vi "Exit Initialize (User).vi"(8 "error in":errorcluster, 11 "Node in":refnum<class "BLS Power Supply Template.lvclass">) -> (0 "error out":errorcluster, 3 "Node out":refnum<class "BLS Power Supply Template.lvclass">)   [LabVIEW 2023, in "BLS Power Supply Template.lvlib" / "BLS Power Supply Template.lvclass"]
uses:
  BLS Power Supply Template.lvclass
  Support/Class/RMXPowerSupply.lvclass
  9af2f5ac-29fe-43a3-9d64-175040de1a66.vi
  Support/Class/RMX4120_Class/RMX4120.lvclass
  D:/git/bls-power-supply-plugin-template/src/Support/Class/RMXPowerSupply.lvclass
  D:/git/bls-power-supply-plugin-template/src/Support/Class/RMX4120_Class/RMX4120.lvclass
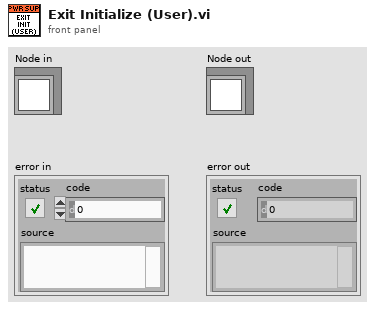
[diagram p1: front panel]
types:
  T1 = typedef "BLS Power Supply Template.lvlib/BLS Power Supply Template.lvclass/Configuration Params.ctl" = cluster{"Common":T2, "Address":string, "RMX Type":string, "Config":string}
  T2 = typedef "Template Node.lvlib/Template Node.lvclass/Common Configuration Params.ctl" = cluster{"Iteration Interval (s)":dbl, "T0 (ns)":u64, "Priority":i32, "Processor":i32, "Wait in Ready State":bool}
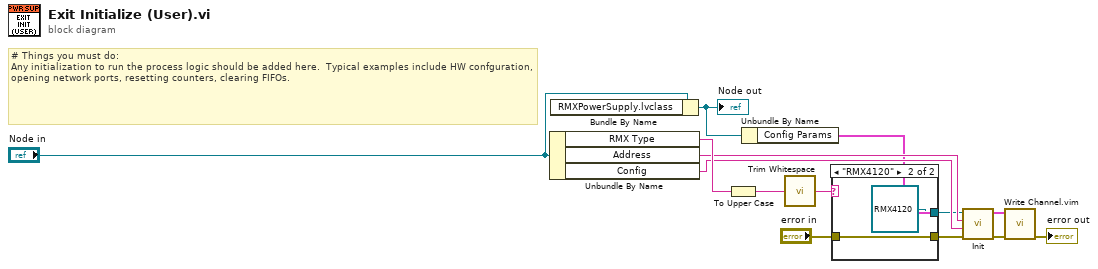
[diagram p0: block diagram]
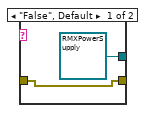
[diagram p2: hidden frame]
diagram:
  # "# Things you must do:\nAny initialization to run the process logic should be added here.  Typical examples include HW confguration, opening network ports, resetting counters, clearing FIFOs."
  n1 = Unbundle By Name("Node in") -> ("RMX Type"=w10:string, "Address"=w9:string, "Config"=w8:string)
  n2 = Bundle By Name(cluster="Node in") -> (w5:refnum<class "BLS Power Supply Template.lvclass">)  [unwired: 1 in]
  "Node out" <- w5
  n3 = To Upper Case(1:w10) -> (0:w12:string)
  n4 = Unbundle By Name(w5) -> ("Config Params"=w1:T1)
  n5 = call <vilib>:"Trim Whitespace.vi"("string"=w12) -> ("trimmed string"=w11:string)  [unwired: 1 in]
  n6 = case shown="\"RMX4120\"" w11 {
    tunnel: [refnum<class "RMXPowerSupply.lvclass"> refnum ("RMXPowerSupply.lvclass") refnum<class "RMX4120.lvclass"> refnum ("RMX4120.lvclass")] -> w7
    tunnel: [w14 w16] -> w4
    tunnel: "error in" -> [w14 w16]
    frame "False", Default {
    }
    frame "RMX4120" {
    }
  }
  n7 = call-dynamic "Init.vi"("error in (no error)"=w4, "ConfigurationJSON"=w8, "Address"=w9, "RMXPowerSupply in"=w7) -> ("error out"=w3:errorcluster)  [unwired: 3 in, 4 out]
  n8 = call "Write Channel.vim"("error in"=w3, "ADAS HIL Channel in"=w1) -> ("error out"=→"error out":errorcluster)  [unwired: 7 in, 2 out]
